vi "Query All Types.vi"(6 "timeout (ms)":i32=5000, 8 "error in":errorcluster, 11 "gRPC ID in":T3) -> (0 "error out":errorcluster, 2 "plugin_types":T1[](array[typedef]), 3 "gRPC ID out":T3)   [LabVIEW 2021, in "CIFManagerClientWrapper.lvlib"]
uses:
  <vilib>/gRPC/LabVIEW gRPC Library/Shared/grpcId.ctl
  CIF_Manager_client/RPC Messages/cif_manager_Empty.ctl
  CIFManagerClientWrapper.lvlib
  CIF_Manager_client/CIF_Manager_client.lvlib
  <vilib>/gRPC/LabVIEW gRPC Library/grpc-lvsupport-release.lvlib
  CIF_Manager_client/RPC Messages/cif_manager_PluginVersion.ctl
  CIF_Manager_client/RPC Messages/cif_manager_PluginType.ctl
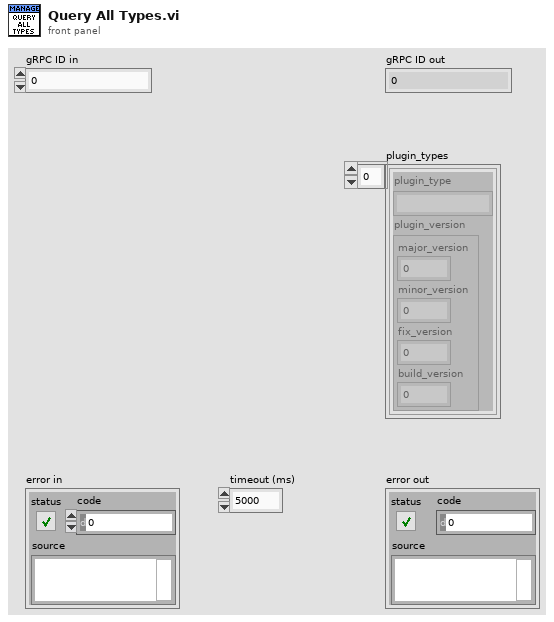
[diagram p1: front panel]
types:
  T1 = typedef "CIF_Manager_client.lvlib/cif_manager_PluginType.ctl" = cluster{"plugin_type":string, "plugin_version":T2}
  T2 = typedef "CIF_Manager_client.lvlib/cif_manager_PluginVersion.ctl" = cluster{"major_version":i32, "minor_version":i32, "fix_version":i32, "build_version":i32}
  T3 = typedef "grpc-lvsupport-release.lvlib/grpcId.ctl" = u64
  T4 = typedef "CIF_Manager_client.lvlib/cif_manager_Empty.ctl" = cluster{"void":string}
  T5 = typedef "CIF_Manager_client.lvlib/cif_manager_PluginTypeReply.ctl" = cluster{"plugin_types":T1[]}
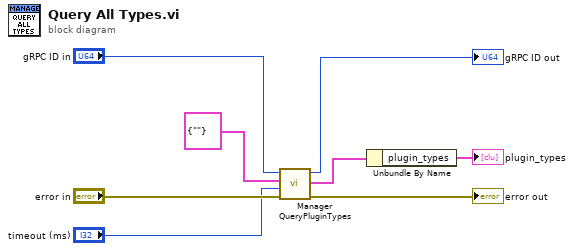
[diagram p0: block diagram]
diagram:
  n1 = call "Manager QueryPluginTypes.vi"("error in"="error in", "timeout (ms)"="timeout (ms)", "Request Data"=T4 {"void"=""}, "gRPC ID"="gRPC ID in") -> ("error out"=→"error out":errorcluster, "Response Data"=w4:T5, "gRPC ID out"=→"gRPC ID out":T3)  [unwired: 5 in]
  n2 = Unbundle By Name(w4) -> ("plugin_types"=→"plugin_types":T1[])
